vi "_testDialogs.vi"() -> ()   [LabVIEW 2012]
uses:
  MessageBox/pictures/pictures.ctl
  ImageGallery/Shuffle time.ctl
  Dialog/Dialog/Dialog.lvclass
  SubPanel/Dummy SubPanel.vi
  Dialog_TwoButtons/Dialog_TwoButtons/Dialog_TwoButtons.lvclass
  MessageBox/MessageBox.lvclass
  Msg_Error/Msg_Error.lvclass
  ImageGallery/Image Gallery.lvclass
  SubPanel/SubPanel.lvclass
panel:
  in  "Shuffle time (5 s)":T1=enum."5s"
  in  "Path to directory":path=path "C:/Users/normandinf/Desktop/test"
  in  "Image path":T2
  in  "Error":errorcluster={"status"=TRUE, "code"=4585, "source"="Test Error Message Box"}
  in  "Timeout (-1)":i32=-1
  in  "Allow to close? (T)":bool=TRUE
  in  "Button #2 text (Cancel)":string="Cancel"
  in  "Button #1 text (OK)":string="OK"
  out "Selection":string
  in  "Show":bool
  in  "Message":string
  in  "Title":string
  in  "Dialog type":T3(ring)
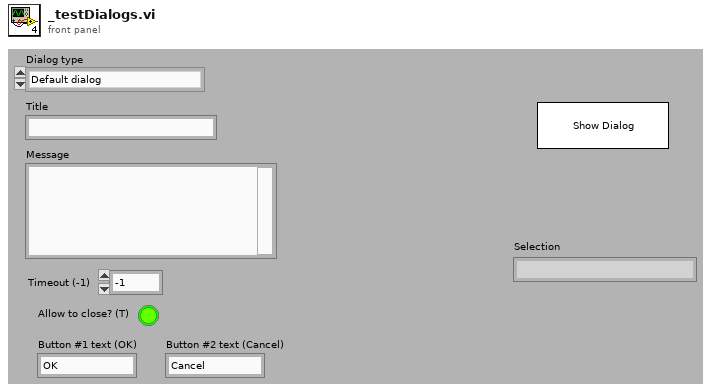
[diagram p1: front panel]
types:
  T1 = typedef "ImageGallery.lvlib/Image Gallery.lvclass/Shuffle time.ctl" = enum16{"Unlimited", "1s", "2s", "3s", "4s", "5s", "7s", "10s", "30s"}
  T2 = typedef "pictures.ctl" = enum16{"Alarm", "Download", "Edition", "Encrypted", "Error", "Hardware Information", "Important", "Memory", "Network", "Package", "Password", "Readme", "Search", "System", "USB", "User", "Wireless", "www"}
  T3 = enum16{"Default dialog", "OK+Cancel Dialog", "Message Box (no button)", "Error Msg", "Image Gallery", "SubPanel"}
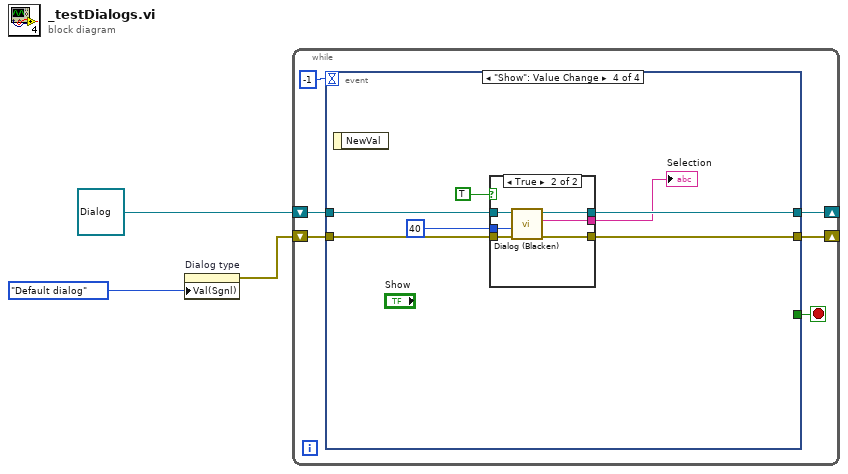
[diagram p0: block diagram]
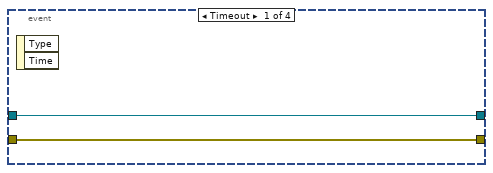
[diagram p2: hidden frame]
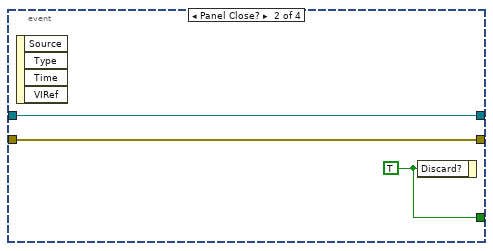
[diagram p3: hidden frame]
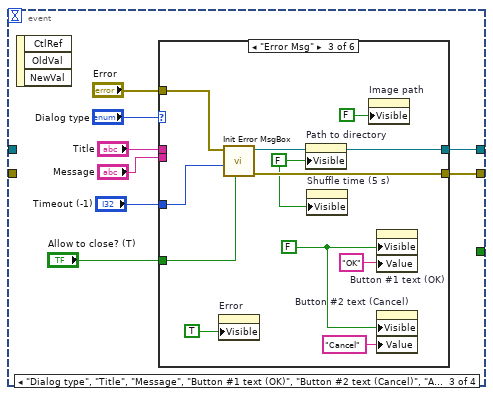
[diagram p4: hidden frame]
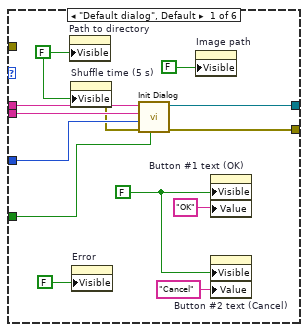
[diagram p5: hidden frame]
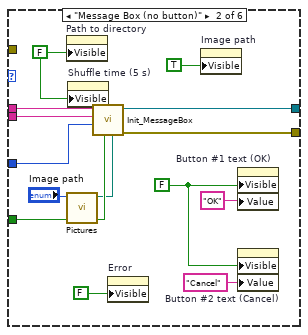
[diagram p6: hidden frame]
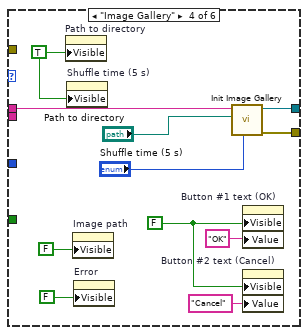
[diagram p7: hidden frame]
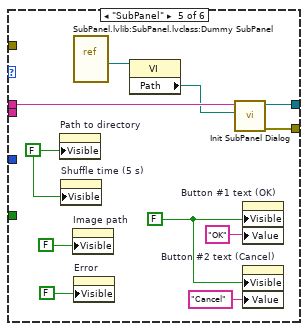
[diagram p8: hidden frame]
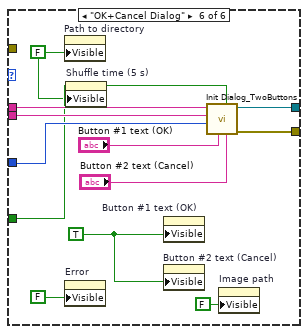
[diagram p9: hidden frame]
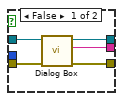
[diagram p10: hidden frame]
diagram:
  n1 = property on="Dialog type" class="Enum (strict)"("Val(Sgnl)"=T3."Default dialog" ("Value (Signaling)")) -> (error out=w2:errorcluster)  [unwired: 2 in, 1 out]
  n2 = while {
    shift-right: [w9] -> _
    shift-left: refnum<class "Dialog.lvclass"> refnum ("Dialog:Dialog.lvclass") -> [w5]
    shift-right: [w8] -> _
    shift-left: w2 -> [w6]
    stop <- w4 stop-if-true
    n3 = event shown="[3] \"Show\": Value Change" {
      selector: _ -> [_ _ _ _]
      dyn-events: _ -> [_ _ _ _]
      timeout: -1 -> [_ _ _ _]
      tunnel: [w10 w13 w19 w100] -> w9
      tunnel: [w11 w14 w18 w99] -> w8
      tunnel: w6 -> [w11 w14 _ w97]
      tunnel: w5 -> [w10 w13 _ w98]
      tunnel: [_ w12 _ _] -> w4
      event Timeout {
        n4 = event-data() -> ()  [unwired: 3 out]
      }
      event Panel Close? {
        w12 = TRUE ("Discard?")
        n5 = event-data() -> ()  [unwired: 5 out]
        n6 = event-data("Discard?"=w12) -> ()  [unwired: 1 in, 1 out]
      }
      event "Dialog type", "Title", "Message", "Button #1 text (OK)", "Button #2 text (Cancel)", "Allow to close? (T)", "Timeout (-1)", "Error", "Path to directory": Value Change {
        n7 = event-data() -> ()  [unwired: 4 out]
        n8 = case shown="\"Error Msg\"" "Dialog type" {
          tunnel: [w30 w47 w57 w66 w77 w91] -> w19
          tunnel: [w29 w46 w56 w65 w76 w90] -> w18
          tunnel: "Message" -> [w31 w45 _ _ _ w92]
          tunnel: "Title" -> [w32 w49 _ w64 w75 w93]
          tunnel: "Timeout (-1)" -> [w28 w48 w55 _ _ w87]
          tunnel: "Allow to close? (T)" -> [w27 w44 w51 _ _ w86]
          tunnel: "Error" -> [_ _ w53 _ _ _]
          frame "Default dialog", Default {
            w24 = FALSE ("Visible")
            w35 = FALSE
            n9 = property on="Path to directory" class="Path"("Visible"=w24) -> ()  [unwired: 2 in, 2 out]
            n10 = property on="Shuffle time (5 s)" class="Enum (strict)"("Visible"=w24) -> (error out=w23:errorcluster)  [unwired: 2 in, 1 out]
            n11 = property on="Error" class="Clust (strict)"("Visible"=FALSE) -> ()  [unwired: 2 in, 2 out]
            n12 = call "Init Dialog.vi"("Allow to close? (T)"=w27, "error in (no error)"=w23, "Timeout (-1)"=w28, "Message"=w31, "Dialog Title"=w32) -> ("error out"=w29:errorcluster, "Dialog out"=w30:refnum<class "Dialog.lvclass">)  [unwired: 1 in, 4 out]
            n13 = property on="Image path" class="Enum (strict)"("Visible"=FALSE) -> ()  [unwired: 2 in, 2 out]
            n14 = property on="Button #1 text (OK)" class="Str"("Visible"=w35, "Value"="OK" ("Button #1 text (OK)")) -> ()  [unwired: 2 in, 2 out]
            n15 = property on="Button #2 text (Cancel)" class="Str"("Visible"=w35, "Value"="Cancel" ("Button #2 text (Cancel)")) -> ()  [unwired: 2 in, 2 out]
          }
          frame "Message Box (no button)" {
            w36 = FALSE ("Visible")
            w43 = FALSE
            n16 = property on="Path to directory" class="Path"("Visible"=w36) -> ()  [unwired: 2 in, 2 out]
            n17 = call "Pictures.vi"("Pictures"="Image path") -> ("Path"=w38:path)  [unwired: 10 out]
            n18 = property on="Shuffle time (5 s)" class="Enum (strict)"("Visible"=w36) -> ()  [unwired: 2 in, 2 out]
            n19 = call "Init_MessageBox.vi"("Image path"=w38, "Allow to close? (T)"=w44, "Timeout (-1)"=w48, "Message"=w45, "MsgBox Title"=w49) -> ("error out"=w46:errorcluster, "MessageBox out"=w47:refnum<class "MessageBox.lvclass">)  [unwired: 2 in, 3 out]
            n20 = property on="Error" class="Clust (strict)"("Visible"=FALSE) -> ()  [unwired: 2 in, 2 out]
            n21 = property on="Image path" class="Enum (strict)"("Visible"=TRUE) -> ()  [unwired: 2 in, 2 out]
            n22 = property on="Button #1 text (OK)" class="Str"("Visible"=w43, "Value"="OK" ("Button #1 text (OK)")) -> ()  [unwired: 2 in, 2 out]
            n23 = property on="Button #2 text (Cancel)" class="Str"("Visible"=w43, "Value"="Cancel" ("Button #2 text (Cancel)")) -> ()  [unwired: 2 in, 2 out]
          }
          frame "Error Msg" {
            w50 = FALSE ("Visible")
            w60 = FALSE
            n24 = property on="Error" class="Clust (strict)"("Visible"=TRUE) -> ()  [unwired: 2 in, 2 out]
            n25 = call "Init Error MsgBox.vi"("Allow to close? (T)"=w51, "Timeout (-1)"=w55, "Error"=w53) -> ("error out"=w56:errorcluster, "Msg_Error out"=w57:refnum<class "Msg_Error.lvclass">)  [unwired: 4 in, 3 out]
            n26 = property on="Path to directory" class="Path"("Visible"=w50) -> ()  [unwired: 2 in, 2 out]
            n27 = property on="Shuffle time (5 s)" class="Enum (strict)"("Visible"=w50) -> ()  [unwired: 2 in, 2 out]
            n28 = property on="Image path" class="Enum (strict)"("Visible"=FALSE) -> ()  [unwired: 2 in, 2 out]
            n29 = property on="Button #1 text (OK)" class="Str"("Visible"=w60, "Value"="OK" ("Button #1 text (OK)")) -> ()  [unwired: 2 in, 2 out]
            n30 = property on="Button #2 text (Cancel)" class="Str"("Visible"=w60, "Value"="Cancel" ("Button #2 text (Cancel)")) -> ()  [unwired: 2 in, 2 out]
          }
          frame "Image Gallery" {
            w61 = TRUE ("Visible")
            w71 = FALSE
            n31 = property on="Path to directory" class="Path"("Visible"=w61) -> ()  [unwired: 2 in, 2 out]
            n32 = property on="Shuffle time (5 s)" class="Enum (strict)"("Visible"=w61) -> ()  [unwired: 2 in, 2 out]
            n33 = property on="Image path" class="Enum (strict)"("Visible"=FALSE) -> ()  [unwired: 2 in, 2 out]
            n34 = property on="Error" class="Clust (strict)"("Visible"=FALSE) -> ()  [unwired: 2 in, 2 out]
            n35 = call "Init Image Gallery.vi"("Shuffle time (5 s)"="Shuffle time (5 s)", "Path to directory"="Path to directory", "ImageGallery Title"=w64) -> ("error out"=w65:errorcluster, "Image Gallery out"=w66:refnum<class "Image Gallery.lvclass">)  [unwired: 3 in, 4 out]
            n36 = property on="Button #1 text (OK)" class="Str"("Visible"=w71, "Value"="OK" ("Button #1 text (OK)")) -> ()  [unwired: 2 in, 2 out]
            n37 = property on="Button #2 text (Cancel)" class="Str"("Visible"=w71, "Value"="Cancel" ("Button #2 text (Cancel)")) -> ()  [unwired: 2 in, 2 out]
          }
          frame "SubPanel" {
            w74 = FALSE ("Visible")
            w82 = FALSE
            n38 = property on="Path to directory" class="Path"("Visible"=w74) -> ()  [unwired: 2 in, 2 out]
            n39 = property on="Shuffle time (5 s)" class="Enum (strict)"("Visible"=w74) -> ()  [unwired: 2 in, 2 out]
            n40 = property on="Image path" class="Enum (strict)"("Visible"=FALSE) -> ()  [unwired: 2 in, 2 out]
            n41 = vi-ref "SubPanel.lvlib:SubPanel.lvclass:Dummy SubPanel.vi"() -> (w73:refnum<vi>)
            n42 = property on="Error" class="Clust (strict)"("Visible"=FALSE) -> ()  [unwired: 2 in, 2 out]
            n43 = property class="VI"(reference=w73) -> ("Path"=w72:path)  [unwired: 1 in, 2 out]
            n44 = call "Init SubPanel Dialog.vi"("VI Path"=w72, "MsgBox Title"=w75) -> ("error out"=w76:errorcluster, "SubPanel out"=w77:refnum<class "SubPanel.lvclass">)  [unwired: 2 in, 6 out]
            n45 = property on="Button #1 text (OK)" class="Str"("Visible"=w82, "Value"="OK" ("Button #1 text (OK)")) -> ()  [unwired: 2 in, 2 out]
            n46 = property on="Button #2 text (Cancel)" class="Str"("Visible"=w82, "Value"="Cancel" ("Button #2 text (Cancel)")) -> ()  [unwired: 2 in, 2 out]
          }
          frame "OK+Cancel Dialog" {
            w83 = FALSE ("Visible")
            w94 = TRUE
            n47 = property on="Path to directory" class="Path"("Visible"=w83) -> ()  [unwired: 2 in, 2 out]
            n48 = property on="Error" class="Clust (strict)"("Visible"=FALSE) -> ()  [unwired: 2 in, 2 out]
            n49 = property on="Shuffle time (5 s)" class="Enum (strict)"("Visible"=w83) -> ()  [unwired: 2 in, 2 out]
            n50 = property on="Button #1 text (OK)" class="Str"("Visible"=w94) -> ()  [unwired: 2 in, 2 out]
            n51 = property on="Button #2 text (Cancel)" class="Str"("Visible"=w94) -> ()  [unwired: 2 in, 2 out]
            n52 = call "Init Dialog_TwoButtons.vi"("Button #2 text (Cancel)"="Button #2 text (Cancel)", "Allow to close? (T)"=w86, "Button #1 text (OK)"="Button #1 text (OK)", "Timeout (-1)"=w87, "Message"=w92, "Dialog Title"=w93) -> ("error out"=w90:errorcluster, "Dialog_2Buttons out"=w91:refnum<class "Dialog_TwoButtons.lvclass">)  [unwired: 2 in, 2 out]
            n53 = property on="Image path" class="Enum (strict)"("Visible"=FALSE) -> ()  [unwired: 2 in, 2 out]
          }
        }
      }
      event "Show": Value Change {
        n54 = event-data() -> ()  [unwired: 2 out]
        n55 = case shown="True" TRUE {
          tunnel: u8 40 ("Transparency (20)") -> [_ w112]
          tunnel: [w103 w111] -> w100
          tunnel: [w102 w110] -> w99
          tunnel: w98 -> [w106 w109]
          tunnel: w97 -> [w105 w108]
          tunnel: [w104 w107] -> w96
          frame False {
            n56 = call-dynamic "Dialog Box.vi"("error in (no error)"=w105, "Dialog in"=w106) -> ("error out"=w102:errorcluster, "Selection"=w104:string, "Dialog out"=w103:refnum<class "Dialog.lvclass">)  [unwired: 7 out]
          }
          frame True {
            n57 = call-dynamic "Dialog (Blacken).vi"("error in (no error)"=w108, "Transparency (40)"=w112, "Dialog in"=w109) -> ("error out"=w110:errorcluster, "Selection"=w107:string, "Dialog out"=w111:refnum<class "Dialog.lvclass">)  [unwired: 6 out]
          }
        }
        "Selection" <- w96
      }
    }
  }
